vi "Read DeviceID.vi"(11 "Device DDS Communications in":refnum<class "Device DDS Communications.lvclass">) -> (2 "DeviceID":T1[](array[typedef]), 3 "Device DDS Communications out":refnum<class "Device DDS Communications.lvclass">)   [LabVIEW 2018, in "Device DDS Communications Framework.lvlib" / "Device DDS Communications.lvclass"]
uses:
  Device DDS Communications.lvclass
  <vilib>/ORNL/CSEISMIC DDS/CSEISMIC DDS Base/Data Types/Controls/DeviceID.ctl
  Device DDS Communications.lvclass/Device DDS Communications.ctl
  <vilib>/ORNL/CSEISMIC DDS/CSEISMIC DDS Base/CSEISMIC DDS.lvclass
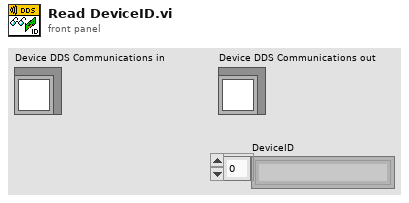
[diagram p1: front panel]
types:
  T1 = typedef "CSEISMIC DDS.lvlib/CSEISMIC DDS.lvclass/DeviceID.ctl" = string
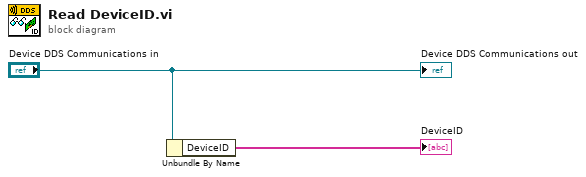
[diagram p0: block diagram]
diagram:
  n1 = Unbundle By Name("Device DDS Communications in") -> ("DeviceID"=→"DeviceID":T1[])
  "Device DDS Communications out" <- "Device DDS Communications in"
